vi "Write Configuration File.vi"(8 "error in (no error)":errorcluster, 11 "Instrument in":refnum<class "Instrument.lvclass">) -> (0 "error out":errorcluster, 3 "Instrument out":refnum<class "Instrument.lvclass">)   [LabVIEW 2019, in "Instrument.lvlib" / "Instrument.lvclass"]
uses:
  Instrument.lvclass
  C:/Program Files (x86)/National Instruments/LabVIEW 2019/vi.lib/JKI/JKI SMO/SMO/SMO.lvclass
  Instrument.lvclass/Instrument.ctl
  <userlib>/LevyLab/Configuration/Configuration.lvclass/Configuration.ctl
  <userlib>/LevyLab/Configuration/Write Section.vi
  <vilib>/JKI/JKI SMO/SMO/Protected/ThisLevelClassName.vi
  <userlib>/LevyLab/Configuration/Configuration.lvclass
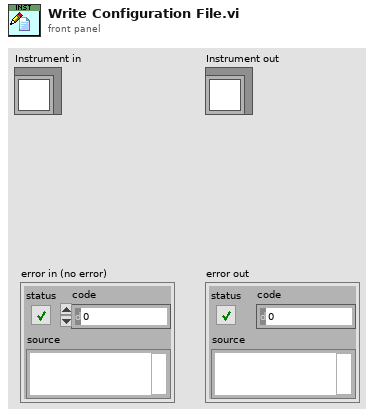
[diagram p1: front panel]
types:
  T1 = typedef "Instrument.lvlib/Instrument.lvclass/Configuration--Cluster.ctl" = cluster{"Hardware":T2, "SMO":T3}
  T2 = typedef "Instrument.lvlib/Instrument.lvclass/HW Configuration--Cluster.ctl" = cluster{"address":string, "type":string}
  T3 = typedef "Instrument.lvlib/Instrument.lvclass/SMO Configuration--Cluster.ctl" = cluster{"Address":string, "Port":u16, "RC Type":T4, "Client Type":T5}
  T4 = typedef "RemoteControl.lvlib/RemoteControl.lvclass/RC Com Type--enum.ctl" = enum16{"RC", "STM", "ZMQ"}
  T5 = typedef "Instrument.lvlib/Instrument.lvclass/Client Type--Enum.ctl" = enum16{"Remote", "Local"}
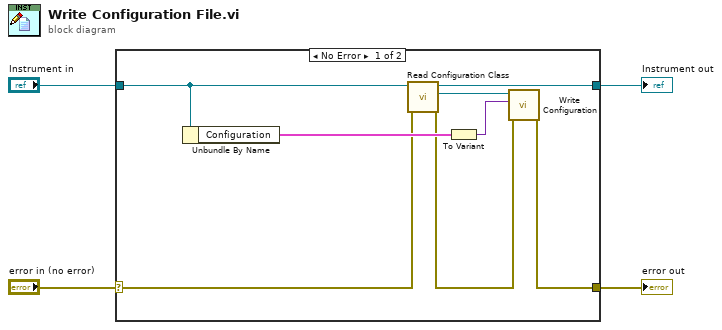
[diagram p0: block diagram]
diagram:
  n1 = case shown="No Error" "error in (no error)" {
    selector: "error in (no error)" -> [w7 w14]
    tunnel: [w12 w13] -> w4
    tunnel: [w10 w14] -> w3
    tunnel: "Instrument in" -> [w8 w13]
    frame No Error {
      n2 = Unbundle By Name(w8) -> ("Configuration"=w9:T1)
      n3 = call "Read Configuration Class.vi"("error in (no error)"=w7, "Instrument in"=w8) -> ("error out"=w6:errorcluster, "Configuration"=w11:refnum<class "Configuration.lvclass">, "Instrument out"=w12:refnum<class "Instrument.lvclass">)  [unwired: 7 in]
      n4 = To Variant(anything=w9) -> (Variant=w5:variant)
      n5 = call <userlib>:"Write Configuration.vi"("error in (no error)"=w6, "Variant"=w5, "Configuration in"=w11) -> ("error out"=w10:errorcluster)  [unwired: 7 in, 1 out]
    }
    frame Error {
    }
  }
  "Instrument out" <- w4
  "error out" <- w3
